vi "Run.vi"(8 "error in (no error)":errorcluster, 11 "PolledDriver in":refnum<class "PolledDriver.lvclass">) -> (0 "error out":errorcluster, 3 "PolledDriver out":refnum<class "PolledDriver.lvclass">)   [LabVIEW 2025, in "PolledDriver.lvclass"]
doc: "This is the main loop of the driver.\nAfter setting up your driver, call this VI to actually run it."
uses:
  PolledDriver.lvclass
  PolledDriver.lvclass/PolledDriver.ctl
  BaseDriver/Read Input queue.vi
  global_stop.vi
  Message/BaseMessage/BaseMessage.lvclass
  BaseDriver/BaseDriver.lvclass
panel:
  out "quit?":bool
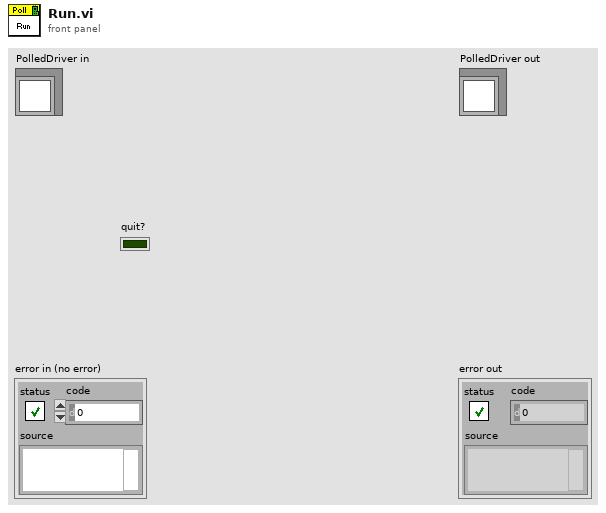
[diagram p1: front panel]
types:
  T1 = typedef "message_queue.ctl" = refnum<queue>
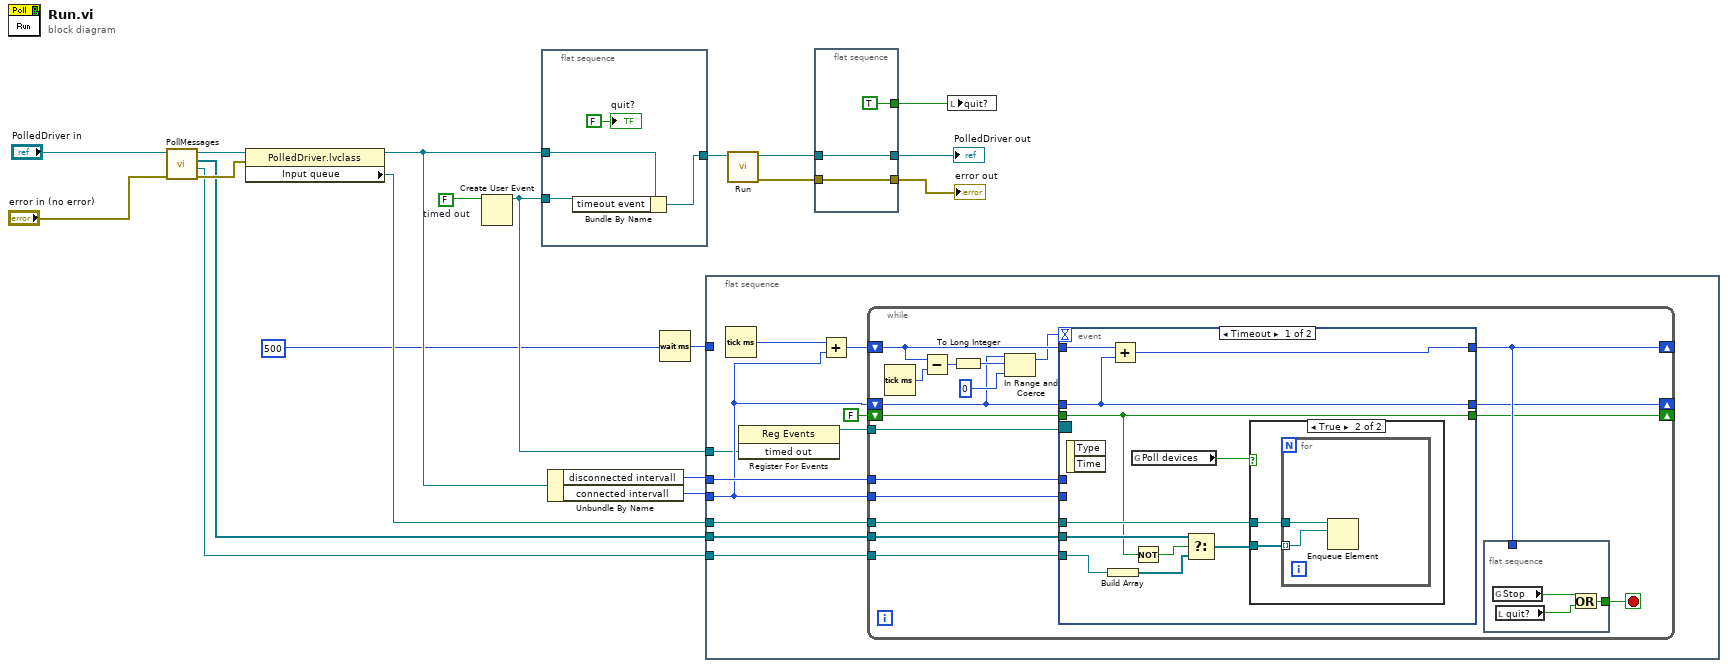
[diagram p0: block diagram]
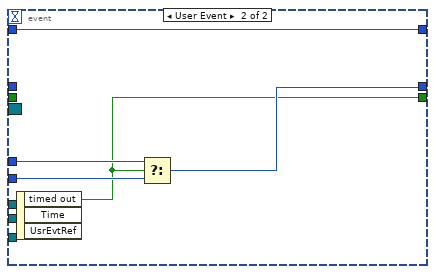
[diagram p3: hidden frame]
diagram:
  w20 = FALSE  # timed out
  n1 = call-dynamic "PollMessages.vi"("error in (no error)"="error in (no error)", "PolledDriver in"="PolledDriver in") -> ("error out"=w8:errorcluster, "disconnected"=w7:refnum<class "BaseMessage.lvclass">, "connected"=w6:refnum<class "BaseMessage.lvclass">[], "PolledDriver out"=w10:refnum<class "PolledDriver.lvclass">)  [unwired: 6 in]
  n2 = property on="Property Node" class="PolledDriver.lvclass"(reference=w10, error in=w8) -> (reference out=w12:refnum<class "PolledDriver.lvclass">, "Input queue"=w5:T1)  [unwired: 1 out]
  n3 = Create User Event(user event datatype=w20) -> (user event=w4:refnum<user-event>)  [unwired: 1 in, 1 out]
  n4 = flat-sequence {
    tunnel: w12 -> [w24]
    tunnel: w4 -> [w23]
    tunnel: [w22] -> w19
    frame #0 {
      n5 = Bundle By Name(cluster=w24, "timeout event"=w23) -> (w22:refnum<class "PolledDriver.lvclass">)
      "quit?" <- FALSE ("quit?")
    }
  }
  n6 = Unbundle By Name(w12) -> ("disconnected intervall"=w3:i32, "connected intervall"=w13:i32)
  n7 = Wait (ms)(milliseconds to wait=u32 500 ("Wait before poll (ms)")) -> (millisecond timer value=w2:u32)
  n8 = flat-sequence {
    tunnel: w4 -> [w25]
    tunnel: w3 -> [w31]
    tunnel: w13 -> [w30]
    tunnel: w7 -> [w26]
    tunnel: w6 -> [w27]
    tunnel: w5 -> [w28]
    tunnel: w2 -> [_]
    frame #0 {
      n9 = Tick Count (ms)() -> (millisecond timer value=w32:u32)
      n10 = register-events(w25) -> (reference out=w34:refnum<event-registration>)  [unwired: 2 in, 1 out]
      n11 = Add(x=w32, y=w30) -> (x+y=w33:u32)
      n12 = while {
        tunnel: w34 -> [w52]
        shift-right: [w44] -> _
        shift-left: w33 -> [w50]
        shift-right: [w41] -> _
        shift-left: w30 -> [w40]
        tunnel: w31 -> [w43]
        tunnel: w30 -> [w42]
        shift-right: [w39] -> _
        shift-left: FALSE ("timed out") -> [w38]
        tunnel: w28 -> [w37]
        tunnel: w27 -> [w36]
        tunnel: w26 -> [w35]
        stop <- w45 stop-if-true
        n13 = Tick Count (ms)() -> (millisecond timer value=w51:u32)
        n14 = Subtract(x=w50, y=w51) -> (x-y=w49:u32)
        n15 = To Long Integer(number=w49) -> (32bit integer=w48:i32)
        n16 = In Range and Coerce(upper limit=w40, x=w48, lower limit=0) -> (coerced(x)=w46:i32)  [unwired: 1 out]
        n17 = event shown="[0] Timeout" {
          selector: w52 -> [_ _]
          dyn-events: _ -> [_ _]
          timeout: w46 -> [_ _]
          tunnel: w50 -> [w66 w75]
          tunnel: [w65 w75] -> w44
          tunnel: w40 -> [w64 _]
          tunnel: w43 -> [_ w74]
          tunnel: w42 -> [_ w73]
          tunnel: [w64 w72] -> w41
          tunnel: [w60 w71] -> w39
          tunnel: w38 -> [w60 _]
          tunnel: w37 -> [w63 _]
          tunnel: w36 -> [w62 _]
          tunnel: w35 -> [w61 _]
          event Timeout {
            n18 = event-data() -> ()  [unwired: 1 in, 2 out]
            n19 = Build Array(w61) -> (w57:refnum<class "BaseMessage.lvclass">[])
            n20 = Add(x=w66, y=w64) -> (x+y=w65:u32)
            n21 = global read "global_stop.vi" "Poll devices"() -> (w56:bool)
            n22 = Not(x=w60) -> (.not. x?=w58:bool)
            n23 = Select(t=w62, s=w58, f=w57) -> (s? t:f=w59:refnum<class "BaseMessage.lvclass">[])
            n24 = case shown="True" w56 {
              tunnel: w63 -> [_ w68]
              tunnel: w59 -> [_ w67]
              frame False {
              }
              frame True {
                n25 = for {
                  tunnel: w68 -> [w70]
                  tunnel: w67 -> [w69] mode=indexing
                  n26 = Enqueue Element(queue=w70, element=w69) -> ()  [unwired: 2 in, 3 out]
                }
              }
            }
          }
          event User Event {
            n27 = event-data() -> ("timed out"=w71:bool)  [unwired: 1 in, 2 out]
            n28 = Select(t=w74, s=w71, f=w73) -> (s? t:f=w72:i32)
          }
        }
        n29 = flat-sequence {
          tunnel: [w55] -> w45
          tunnel: w44 -> [_]
          frame #0 {
            n30 = global read "global_stop.vi" "Stop"() -> (w54:bool)
            n31 = local read "quit?"() -> (w53:bool)
            n32 = Or(x=w54, y=w53) -> (x .or. y?=w55:bool)
          }
        }
      }
    }
  }
  n33 = call-parent "Run.vi"("BaseDriver in"=w19) -> ("error out"=w15:errorcluster, "BaseDriver out"=w17:refnum<class "PolledDriver.lvclass">)  [unwired: 9 in]
  n34 = flat-sequence {
    tunnel: [w78] -> w18
    tunnel: w17 -> [w78]
    tunnel: [w77] -> w16
    tunnel: w15 -> [w77]
    tunnel: [TRUE ("quit?")] -> w14
    frame #0 {
    }
  }
  n35 = local write "quit?"(w14) -> ()
  "error out" <- w16
  "PolledDriver out" <- w18
